vi "LPC2468_Interrupt_Template.vi"(10 "param":u32, 11 "vector":T1(ring)=enum."Timer 1") -> ()   [LabVIEW 2011]
doc: "Interrupt template for LabVIEW Embedded targets. This handler VI can be used to handle all interrupts (or it can be duplicated for each interrupt)."
panel:
  # "This VI will run as an interrupt service routine."
  # "vector indentifies the interrupt vector number for the interrupt."
  # "param is always zero for this target but is a necessary component of the interrupt VI connector pane. To avoid code generation errors, you must leave the param control on the front panel and in the connector pane."
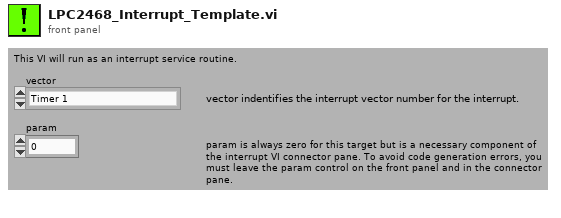
[diagram p1: front panel]
types:
  T1 = enum32{"Unused 0", "Unused 1", "Unused 2", "Unused 3", "Unused 4", "Timer 1", "Unused 6", "Unused 7", "Unused 8", "Unused 9", "Unused 10", "Unused 11", "Unused 12", "Unused 13", "External 0", "External 1", "External 2", "External 3", "Unused 18", "Unused 19", "Unused 20", "Unused 21", "Unused 22", "Unused 23", "Unused 24", "Unused 25", "Timer 2", "Timer 3"}
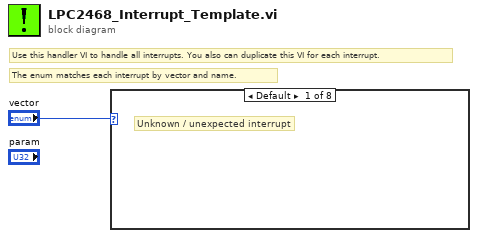
[diagram p0: block diagram]
diagram:
  # "The enum matches each interrupt by vector and name."
  # "Use this handler VI to handle all interrupts. You also can duplicate this VI for each interrupt."
  n1 = case shown="Default" "vector" {
    frame Default {
      # "Unknown / unexpected interrupt"
    }
    frame "Timer 1" {
    }
    frame "External 0" {
    }
    frame "External 1" {
    }
    frame "External 2" {
    }
    frame "External 3" {
    }
    frame "Timer 2" {
    }
    frame "Timer 3" {
    }
  }
